vi "Init.vi"(6 "Export Data To":string="Export Data To", 7 "Prepend Result Name":bool, 8 "error in (no error)":errorcluster, 9 "Test Data Source":string="Test Data Source", 10 "Test Name":string="Test Name", 11 "Measurement Name":string) -> (0 "error out":errorcluster, 3 "Null_Session out":refnum<class "Null Adapter.lvclass">)   [LabVIEW 2018, in "SeqAuto Evaluations.lvlib" / "Null Adapter.lvclass"]
uses:
  Null Adapter.lvclass
  C:/Sequence Automation/Plugins/SeqAuto IEvaluation.lvlibp/SeqAuto IEvaluation.lvclass
  Plugins/SeqAuto IEvaluation.lvlibp/Write Measurement Name.vi
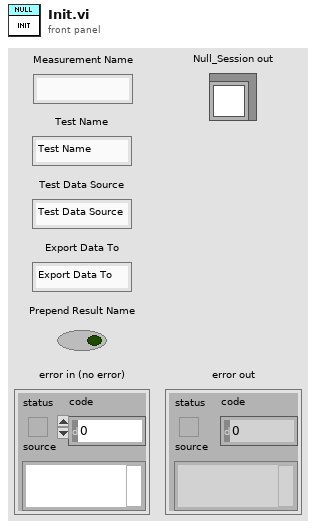
[diagram p1: front panel]
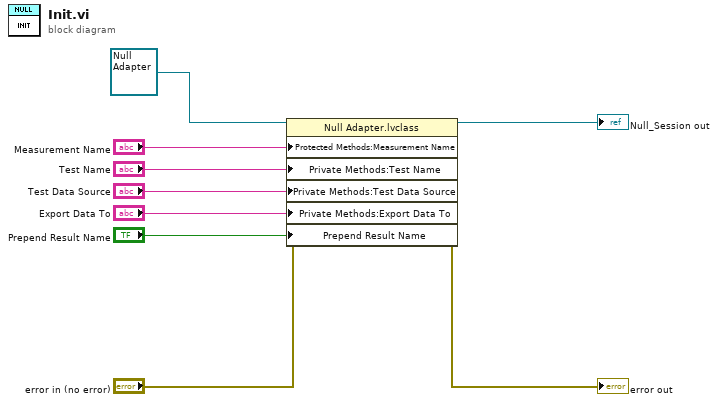
[diagram p0: block diagram]
diagram:
  n1 = property class="Null Adapter.lvclass"(reference=refnum<class "Null Adapter.lvclass"> refnum ("DCLeakage in"), error in="error in (no error)", "Protected Methods:Measurement Name"="Measurement Name", "Private Methods:Test Name"="Test Name", "Private Methods:Test Data Source"="Test Data Source", "Private Methods:Export Data To"="Export Data To", "Prepend Result Name"="Prepend Result Name") -> (reference out=→"Null_Session out":refnum<class "Null Adapter.lvclass">, error out=→"error out":errorcluster)
